vi "where M0 (SubVI).vi"(5 "요구":T1={"국번"="0", "커맨드"="01", "데이터 No."="80"}, 8 "VISA 참조 번호 입력":refnum<visa-resource-name>) -> (0 "x = y?":bool, 2 "숫자 2":i32, 3 "VISA 참조 번호 출력":refnum<visa-resource-name>)   [LabVIEW 2014]
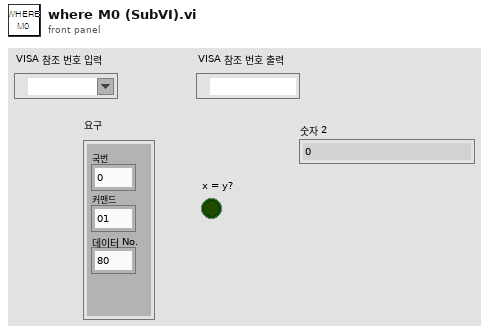
[diagram p1: front panel]
types:
  T1 = cluster{"국번":string, "커맨드":string, "데이터 No.":string}
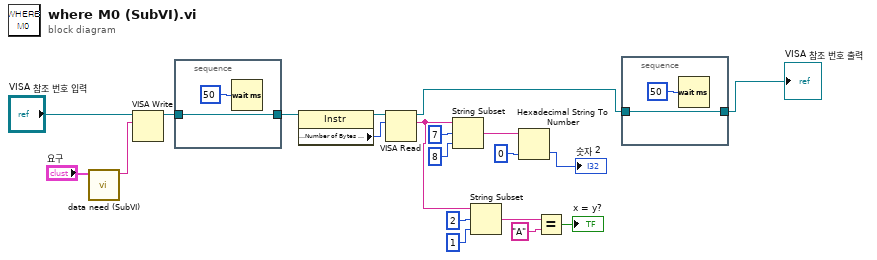
[diagram p0: block diagram]
diagram:
  n1 = call "data need (SubVI).vi"("요구"="요구") -> ("출력"=w17:string)  [unwired: 10 in]
  n2 = VISA Write(VISA resource name="VISA 참조 번호 입력", write buffer=w17) -> (VISA resource name out=w13:refnum<visa-resource-name>)  [unwired: 1 in, 2 out]
  n3 = stacked-sequence {
    tunnel: w13 -> [w22]
    tunnel: [w22] -> w14
    frame #0 {
      n4 = Wait (ms)(milliseconds to wait=u32 50 ("delay before read (ms)")) -> ()  [unwired: 1 out]
    }
  }
  n5 = property on="Property Node" class="Instr"(reference=w14) -> (reference out=w15:refnum<visa-resource-name>, "Serial Settings:Number of Bytes at Serial Port"=w16:u32)  [unwired: 1 in, 1 out]
  n6 = VISA Read(VISA resource name=w15, byte count=w16) -> (VISA resource name out=w2:refnum<visa-resource-name>, read buffer=w4:string)  [unwired: 1 in, 2 out]
  n7 = String Subset(string=w4, offset (0)=7 ("오프셋(0)"), length (rest)=8 ("길이(나머지)")) -> (substring=w20:string)
  n8 = String Subset(string=w4, offset (0)=2 ("오프셋(0)"), length (rest)=1 ("길이(나머지)")) -> (substring=w7:string)
  n9 = Hexadecimal String To Number(string=w20, default (0uL)=0) -> (number=→"숫자 2":i32)  [unwired: 1 in, 1 out]
  n10 = Equal?(x=w7, y="A") -> (x = y?=→"x = y?":bool)
  n11 = stacked-sequence {
    tunnel: w2 -> [w24]
    tunnel: [w24] -> w3
    frame #0 {
      n12 = Wait (ms)(milliseconds to wait=u32 50 ("delay before read (ms)")) -> ()  [unwired: 1 out]
    }
  }
  "VISA 참조 번호 출력" <- w3
